vi "Com_Cmd.vi"(6 "Timeout":i32=1000, 7 "Query":bool, 8 "error in":errorcluster, 9 "Delay, ms":u32=1000, 10 "write buffer":string="PM:P?", 11 "VISA":refnum<visa-resource-name>="COM1") -> (0 "error out":errorcluster, 1 "number":dbl format="%#.6e", 2 "read buffer":string, 3 "VISA Out":refnum<visa-resource-name>, 4 "Timeout":bool, 5 "return count":u32)   [LabVIEW 2017]
panel:
  out "read buffer 2":string
  out "old buffer":string
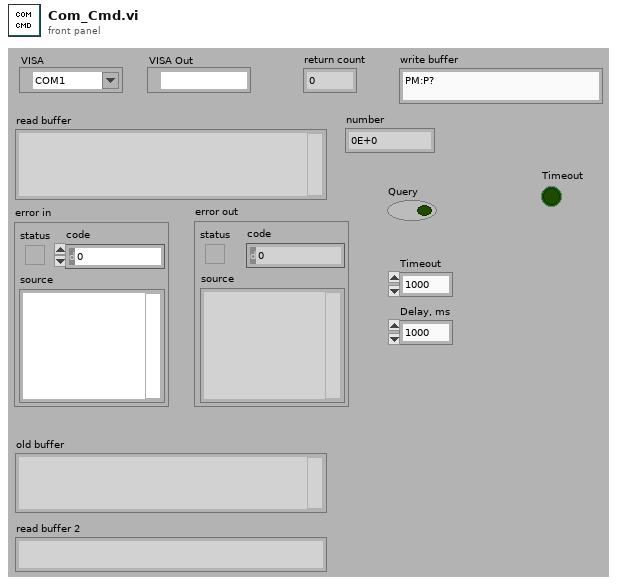
[diagram p1: front panel]
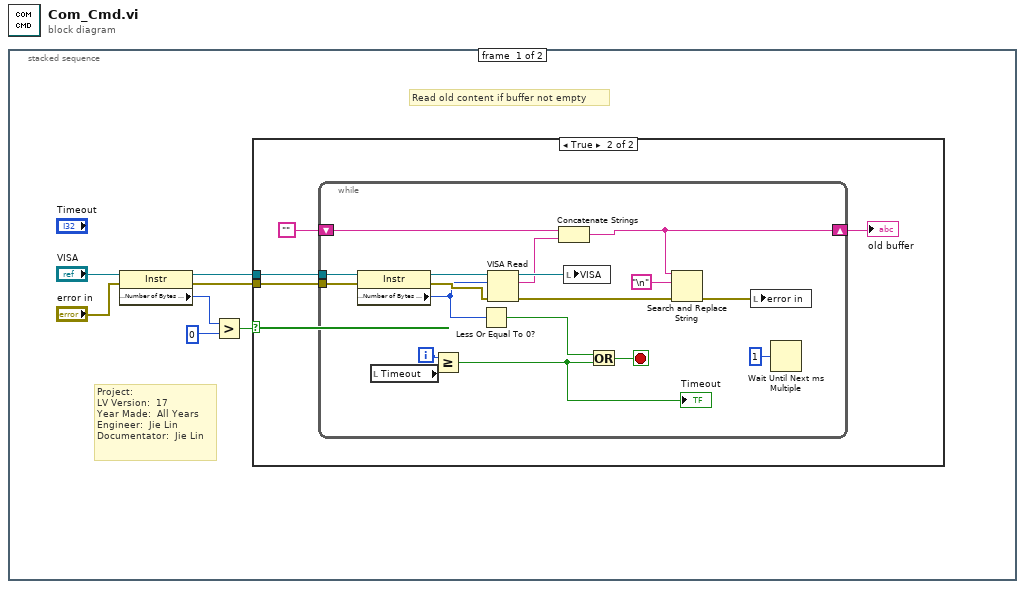
[diagram p0: block diagram]
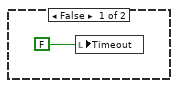
[diagram p2: hidden frame]
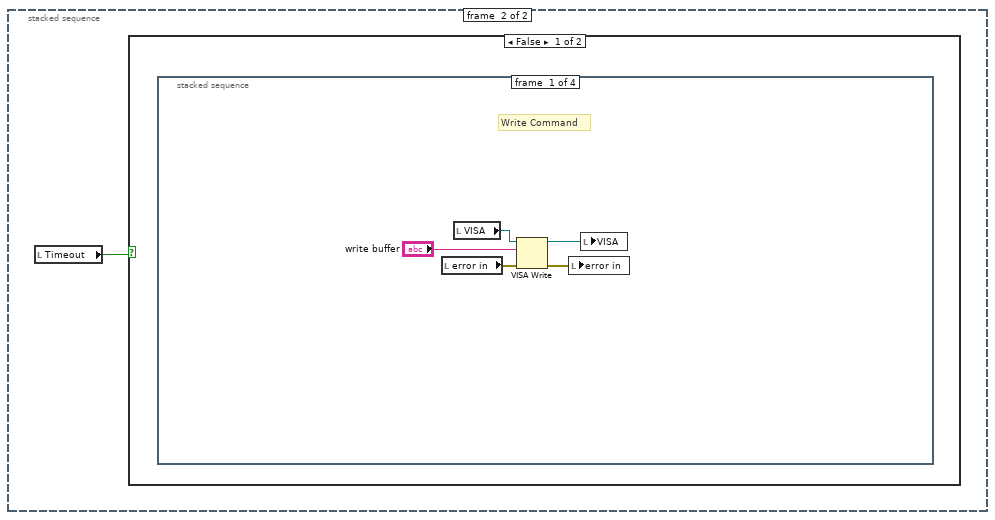
[diagram p3: hidden frame]
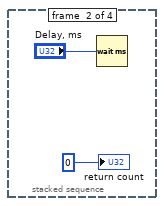
[diagram p4: hidden frame]
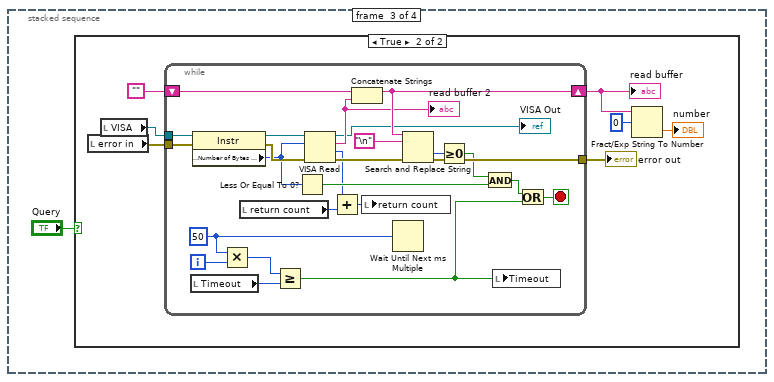
[diagram p5: hidden frame]
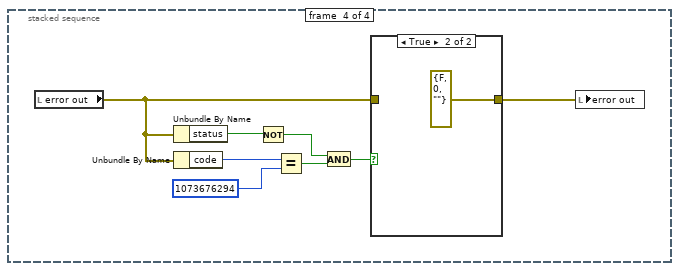
[diagram p7: hidden frame]
diagram:
  n1 = stacked-sequence {
    frame #0 {
      # "Project:  \nLV Version:  17\nYear Made:  All Years\nEngineer:  Jie Lin\nDocumentator:  Jie Lin"
      # "Read old content if buffer not empty"
      n2 = property class="Instr"(reference="VISA", error in="error in") -> (reference out=w2:refnum<visa-resource-name>, error out=w3:errorcluster, "Serial Settings:Number of Bytes at Serial Port"=w4:u32)
      n3 = Greater?(x=w4, y=u32 0) -> (0:w1:bool)
      n4 = case shown="True" w1 {
        tunnel: w3 -> [_ w12]
        tunnel: w2 -> [_ w11]
        frame False {
          n5 = local write "Timeout"(FALSE ("Timeout")) -> ()
        }
        frame True {
          n6 = while {
            tunnel: w12 -> [w16]
            tunnel: w11 -> [w17]
            shift-right: [w26] -> w9
            shift-left: "" -> [w28]
            i -> [w22]
            stop <- w21 stop-if-true
            n7 = property class="Instr"(reference=w17, error in=w16) -> (reference out=w19:refnum<visa-resource-name>, error out=w18:errorcluster, "Serial Settings:Number of Bytes at Serial Port"=w14:u32)
            n8 = local read "Timeout"() -> (w23:i32)
            n9 = Greater Or Equal?(x=w22, y=w23) -> (x >= y?=w13:bool)
            "Timeout" <- w13
            n10 = Less Or Equal To 0?(x=w14) -> (x <= 0?=w24:bool)
            n11 = VISA Read(VISA resource name=w19, byte count=w14, error in (no error)=w18) -> (VISA resource name out=w30:refnum<visa-resource-name>, read buffer=w27:string, error out=w25:errorcluster)  [unwired: 1 out]
            n12 = Concatenate Strings(w28, w27) -> (w26:string)
            n13 = local write "VISA"(w30) -> ()
            n14 = Or(x=w24, y=w13) -> (x .or. y?=w21:bool)
            n15 = Search and Replace String(input string=w26, search string="\n", error in=w25) -> (error out=w20:errorcluster)  [unwired: 5 in, 3 out]
            n16 = local write "error in"(w20) -> ()
            n17 = Wait Until Next ms Multiple(millisecond multiple=u32 1) -> ()  [unwired: 1 out]
          }
          "old buffer" <- w9
        }
      }
    }
    frame #1 {
      n18 = local read "Timeout"() -> (w31:bool)
      n19 = case shown="False" w31 {
        frame False {
          n20 = stacked-sequence {
            frame #0 {
              # "Write Command"
              n21 = local read "error in"() -> (w34:errorcluster)
              n22 = local read "VISA"() -> (w33:refnum<visa-resource-name>)
              n23 = VISA Write(VISA resource name=w33, write buffer="write buffer", error in (no error)=w34) -> (VISA resource name out=w36:refnum<visa-resource-name>, error out=w35:errorcluster)  [unwired: 1 out]
              n24 = local write "error in"(w35) -> ()
              n25 = local write "VISA"(w36) -> ()
            }
            frame #1 {
              n26 = Wait (ms)(milliseconds to wait="Delay, ms") -> ()  [unwired: 1 out]
              "return count" <- u32 0 ("return count")
            }
            frame #2 {
              n27 = case shown="True" "Query" {
                frame False {
                }
                frame True {
                  n28 = local read "error in"() -> (w43:errorcluster)
                  n29 = local read "VISA"() -> (w44:refnum<visa-resource-name>)
                  n30 = while {
                    tunnel: w43 -> [w66]
                    tunnel: w44 -> [w67]
                    shift-right: [w57] -> w42
                    shift-left: "" -> [w71]
                    tunnel: [w63] -> w41
                    i -> [w50]
                    stop <- w68 stop-if-true
                    w49 = u32 50 ("millisecond multiple")
                    n31 = local read "Timeout"() -> (w69:i32)
                    n32 = property class="Instr"(reference=w67, error in=w66) -> (reference out=w65:refnum<visa-resource-name>, error out=w64:errorcluster, "Serial Settings:Number of Bytes at Serial Port"=w62:u32)
                    n33 = Multiply(x=w49, y=w50) -> (x*y=w48:u32)
                    n34 = local read "return count"() -> (w54:u32)
                    n35 = Greater Or Equal?(x=w48, y=w69) -> (x >= y?=w52:bool)
                    n36 = Less Or Equal To 0?(x=w62) -> (x <= 0?=w60:bool)
                    n37 = VISA Read(VISA resource name=w65, byte count=w62, error in (no error)=w64) -> (VISA resource name out=→"VISA Out":refnum<visa-resource-name>, read buffer=w56:string, return count=w55:u32, error out=w70:errorcluster)
                    "read buffer 2" <- w56
                    n38 = Add(x=w55, y=w54) -> (x+y=w53:u32)
                    n39 = Concatenate Strings(w71, w56) -> (w57:string)
                    n40 = local write "return count"(w53) -> ()
                    n41 = Wait Until Next ms Multiple(millisecond multiple=w49) -> ()  [unwired: 1 out]
                    n42 = Search and Replace String(input string=w57, search string="\n", error in=w70) -> (offset past replacement=w58:i32, error out=w63:errorcluster)  [unwired: 5 in, 2 out]
                    n43 = Greater Or Equal To 0?(x=w58) -> (x >= 0?=w61:bool)
                    n44 = And(x=w61, y=w60) -> (x .and. y?=w59:bool)
                    n45 = local write "Timeout"(w52) -> ()
                    n46 = Or(x=w59, y=w52) -> (x .or. y?=w68:bool)
                  }
                  "error out" <- w41
                  "read buffer" <- w42
                  n47 = Fract/Exp String To Number(string=w42, offset=0) -> (number=→"number":dbl)  [unwired: 2 in, 1 out]
                }
              }
            }
            frame #3 {
              n48 = local read "error out"() -> (w72:errorcluster)
              n49 = Unbundle By Name(w72) -> ("status"=w77:bool)
              n50 = Unbundle By Name(w72) -> ("code"=w79:i32)
              n51 = Not(x=w77) -> (.not. x?=w75:bool)
              n52 = Equal?(x=w79, y=1073676294) -> (x = y?=w76:bool)
              n53 = And(x=w75, y=w76) -> (x .and. y?=w74:bool)
              n54 = case shown="True" w74 {
                tunnel: [w80 errorcluster {"status"=FALSE, "code"=0, "source"=""} ("error out")] -> w73
                tunnel: w72 -> [w80 _]
                frame False {
                }
                frame True {
                }
              }
              n55 = local write "error out"(w73) -> ()
            }
          }
        }
        frame True {
        }
      }
    }
  }
